vi "Panel Add New Control.vi"(8 "error in (no error)":errorcluster, 11 "PanelManager in":refnum<class "PanelManager.lvclass">) -> (0 "error out":errorcluster, 3 "PanelManager out":refnum<class "PanelManager.lvclass">)   [LabVIEW 2015, in "PanelManager.lvclass"]
uses:
  PanelManager.lvclass
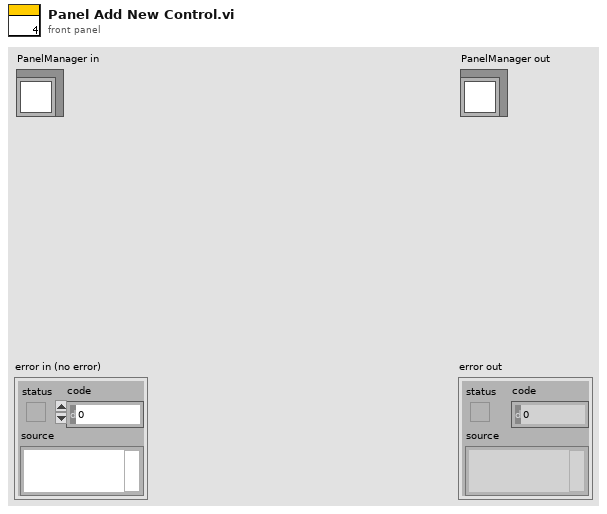
[diagram p1: front panel]
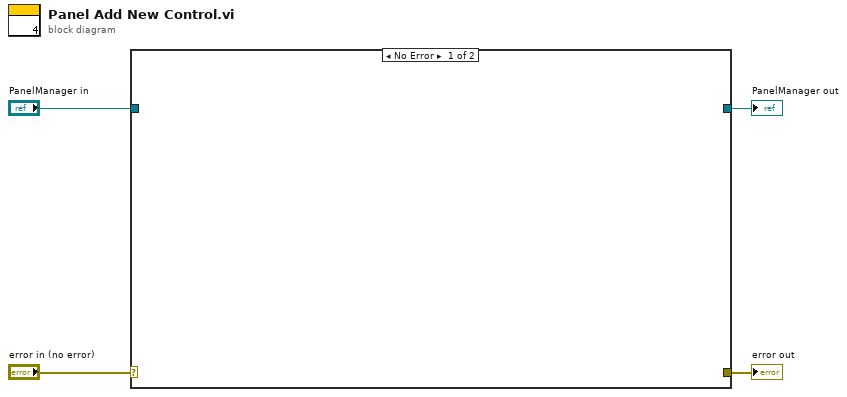
[diagram p0: block diagram]
diagram:
  n1 = case shown="No Error" "error in (no error)" {
    selector: "error in (no error)" -> [_ w6]
    tunnel: [_ w6] -> w3
    tunnel: [_ w5] -> w1
    tunnel: "PanelManager in" -> [_ w5]
    frame No Error {
    }
    frame Error {
    }
  }
  "error out" <- w3
  "PanelManager out" <- w1
